vi "remove start time channel from channel array.vi"(11 "channels in":refnum<class "TBM channel.lvclass">[](array[class])) -> (3 "channels out":refnum<class "TBM channel.lvclass">[](array[class]))   [LabVIEW 2013, in "Shared Memory configuration.lvclass"]
uses:
  Shared Memory configuration.lvclass
  <vilib>/NI/Tag Bus Module Framework/channel/TBM channel.lvclass
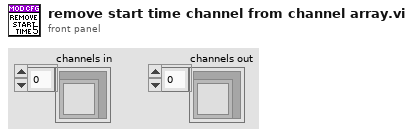
[diagram p1: front panel]
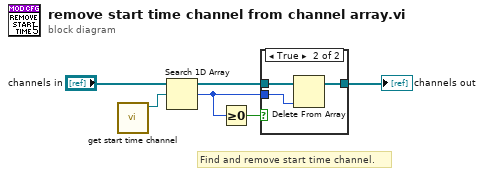
[diagram p0: block diagram]
diagram:
  # "Find and remove start time channel."
  n1 = call "get start time channel.vi"() -> ("channel"=w5:refnum<class "TBM channel.lvclass">)  [unwired: 11 in]
  n2 = Search 1D Array(1D array="channels in", element=w5) -> (index of element=w2:i32)  [unwired: 1 in]
  n3 = Greater Or Equal To 0?(x=w2) -> (x >= 0?=w1:bool)
  n4 = case shown="True" w1 {
    tunnel: "channels in" -> [w6 w9]
    tunnel: [w6 w8] -> w3
    tunnel: w2 -> [_ w7]
    frame False {
    }
    frame True {
      n5 = Delete From Array(array=w9, index=w7) -> (array with subset deleted=w8:refnum<class "TBM channel.lvclass">[])  [unwired: 1 in, 1 out]
    }
  }
  "channels out" <- w3
